vi "add remark(SubVI).vi"() -> (1 "ok or cancel":bool, 2 "连接的字符串":string)   [LabVIEW 2019, in "Add Seq.lvlib"]
uses:
  Add Seq.lvlib
panel:
  in  "分隔符":string
  in  "cancel":bool
  in  "ok":bool
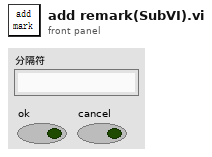
[diagram p1: front panel]
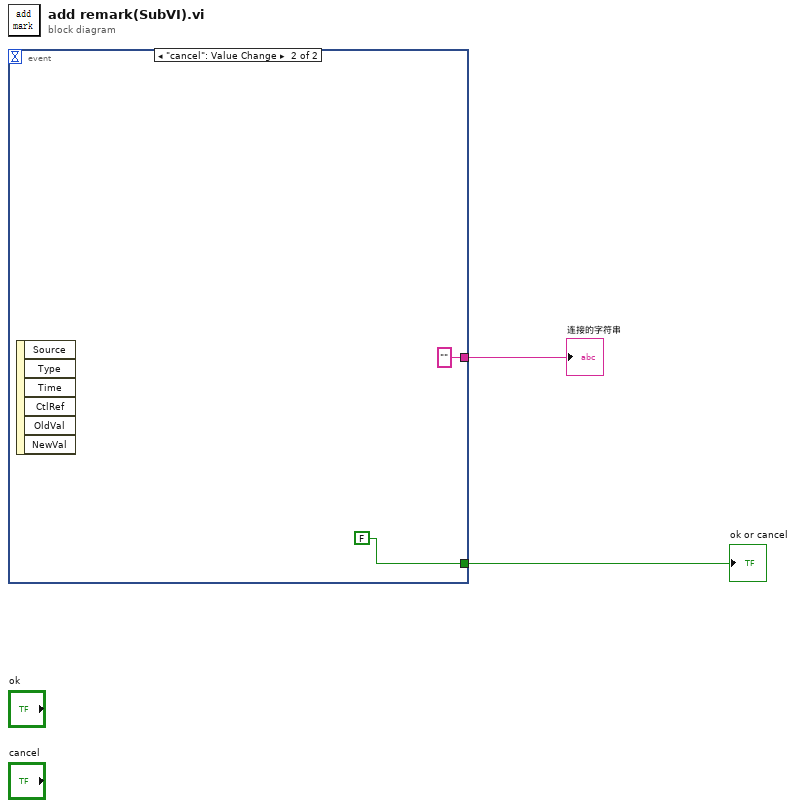
[diagram p0: block diagram]
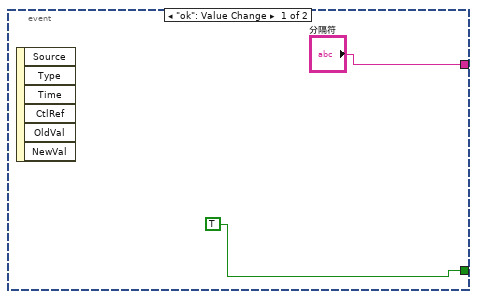
[diagram p2: hidden frame]
diagram:
  n1 = event shown="[1] \"cancel\": Value Change" {
    selector: _ -> [_ _]
    dyn-events: _ -> [_ _]
    timeout: _ -> [_ _]
    tunnel: [TRUE FALSE] -> w2
    tunnel: ["分隔符" "" ("分隔符")] -> w1
    event "ok": Value Change {
      n2 = event-data() -> ()  [unwired: 1 in, 6 out]
    }
    event "cancel": Value Change {
      n3 = event-data() -> ()  [unwired: 1 in, 6 out]
    }
  }
  "ok or cancel" <- w2
  "连接的字符串" <- w1
